vi "Untitled 2.vi"   [LabVIEW 2013]
uses:
  lightfield-automation-labview/VIs/ClientServerMode/CS_LFAClassGlobal.vi
  lightfield-automation-labview/LightField Automation.lvclass
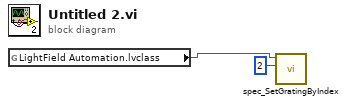
[diagram p0: block diagram]
diagram:
  n1 = global read "CS_LFAClassGlobal.vi" "LightField Automation.lvclass"() -> (w2:refnum<class "LightField Automation.lvclass">)
  n2 = call "spec_SetGratingByIndex.vi"("Grating Index (0 -> n-1)"=2, "LightField Automation in"=w2) -> ()  [unwired: 8 in, 2 out]
